vi "CreateHsimple.vi"(2 "[Y]":dbl[](array[numeric]), 3 "[X]":dbl[](array[numeric]), 4 "Highest order":i32) -> (0 "H":dbl[][](array[numeric]))   [LabVIEW 2011]
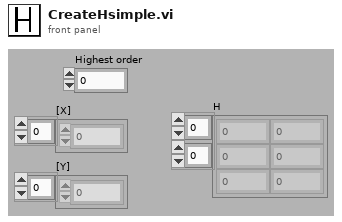
[diagram p1: front panel]
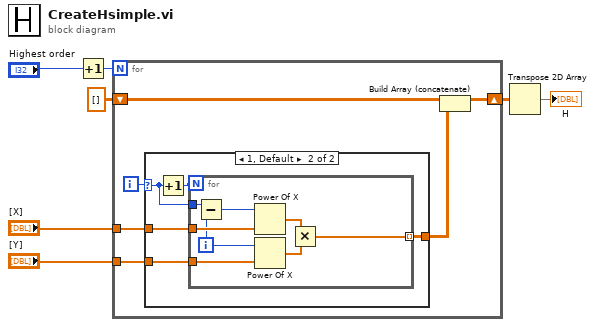
[diagram p0: block diagram]
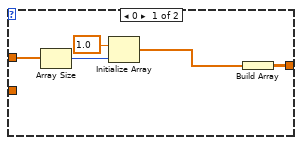
[diagram p2: hidden frame]
diagram:
  n1 = Increment(x="Highest order") -> (x+1=w2:i32)
  n2 = for {
    N: w2 -> [_]
    tunnel: "[X]" -> [w11]
    tunnel: "[Y]" -> [w13]
    shift-right: [w8] -> w7
    shift-left: dbl[][] [] ("transposed array") -> [w9]
    i -> [w12]
    n3 = case shown="1, Default" w12 {
      selector: w12 -> [_ w20]
      tunnel: w13 -> [_ w24]
      tunnel: w11 -> [w18 w23]
      tunnel: [w16 w21] -> w10
      frame 0 {
        n4 = Array Size(array=w18) -> (size(s)=w17:i32)
        n5 = Initialize Array(1.0 ("element"), w17) -> (w15:dbl[])
        n6 = Build Array(w15) -> (w16:dbl[][])
        n7 = Build Array("" ("format string")) -> ()  [unwired: 1 out]
      }
      frame 1, Default {
        n8 = Increment(x=w20) -> (x+1=w22:i32)
        n9 = for {
          N: w22 -> [_]
          tunnel: w24 -> [w32]
          tunnel: w23 -> [w31]
          tunnel: w20 -> [w30]
          tunnel: [w27] -> w21 mode=indexing
          i -> [w25]
          n10 = Subtract(x=w30, y=w25) -> (x-y=w26:i32)
          n11 = Power Of X(1:w31, 2:w26) -> (0:w29:dbl[])
          n12 = Power Of X(1:w32, 2:w25) -> (0:w28:dbl[])
          n13 = Multiply(x=w29, y=w28) -> (x*y=w27:dbl[])
        }
      }
    }
    n14 = Build Array (concatenate)(w9, w10) -> (w8:dbl[][])
  }
  n15 = Transpose 2D Array(2D array=w7) -> (transposed array=→"H":dbl[][])
